vi "Get Key with Raw Name Cacher(inline).vi"(10 "key":string, 11 "namecacher map in":variant) -> (1 "Raw name":string, 2 "Key in lower case":string, 3 "namecacher map out":variant)   [LabVIEW 2017]
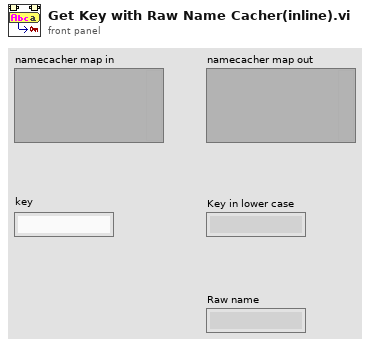
[diagram p1: front panel]
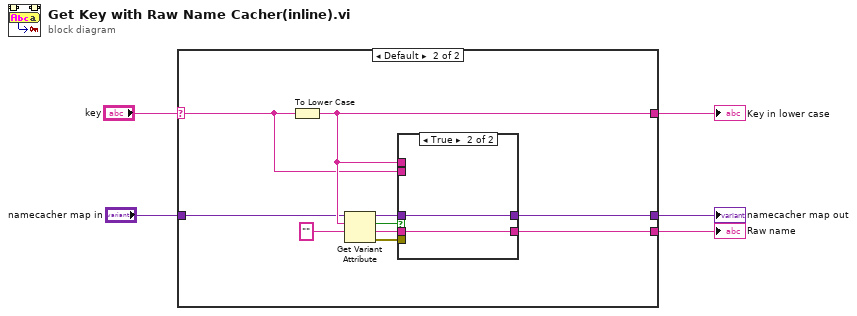
[diagram p0: block diagram]
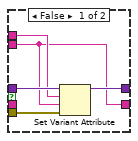
[diagram p3: hidden frame]
diagram:
  n1 = case shown="Default" "key" {
    selector: "key" -> [_ w15]
    tunnel: [_ w16] -> w5
    tunnel: [_ w14] -> w3
    tunnel: [w6 w8] -> w1
    tunnel: "namecacher map in" -> [w6 w7]
    frame "" {
    }
    frame Default {
      n2 = To Lower Case(string=w15) -> (all lower case string=w16:string)
      n3 = Get Variant Attribute(Variant=w7, name=w16, default value (empty Variant)="") -> (duplicate Variant=w13:variant, found=w11:bool, value=w10:string, error out=w9:errorcluster)  [unwired: 1 in]
      n4 = case shown="True" w11 {
        tunnel: w13 -> [w21 w23]
        tunnel: w16 -> [w20 _]
        tunnel: w15 -> [w17 _]
        tunnel: w10 -> [_ w22]
        tunnel: w9 -> [w19 _]
        tunnel: [w18 w23] -> w8
        tunnel: [w17 w22] -> w14
        frame False {
          n5 = Set Variant Attribute(Variant=w21, name=w20, value=w17, error in=w19) -> (Variant out=w18:variant)  [unwired: 2 out]
        }
        frame True {
        }
      }
    }
  }
  "Key in lower case" <- w5
  "Raw name" <- w3
  "namecacher map out" <- w1
